vi "Turn All Outputs Off.vi"(8 "error in":errorcluster, 11 "6700C in":refnum<class "6700C.lvclass">) -> (0 "error out":errorcluster, 3 "6700C out":refnum<class "6700C.lvclass">)   [LabVIEW 2019, in "6700C.lvlib" / "6700C.lvclass"]
uses:
  Library/6700C.lvclass
  C:/Users/Public/Documents/Development/builds/Instruments/PowerSupply.lvlibp/Library/PowerSupply.lvclass
  builds/Instruments/PowerSupply.lvlibp/Private/Accessors/Read Number of Channels.vi
  builds/Instruments/PowerSupply.lvlibp/Accessors/Write Active Channel.vi
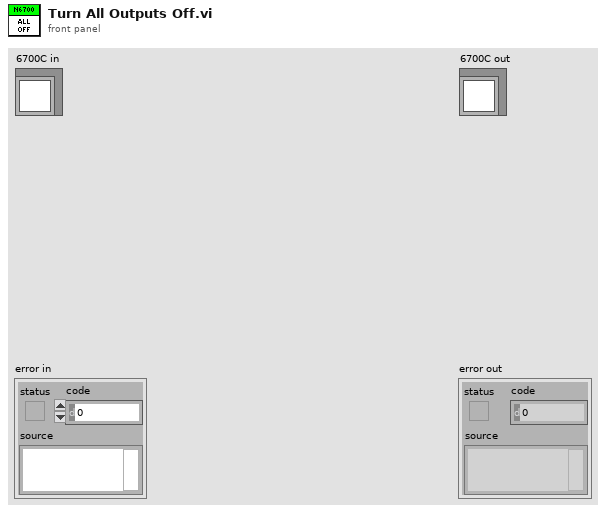
[diagram p1: front panel]
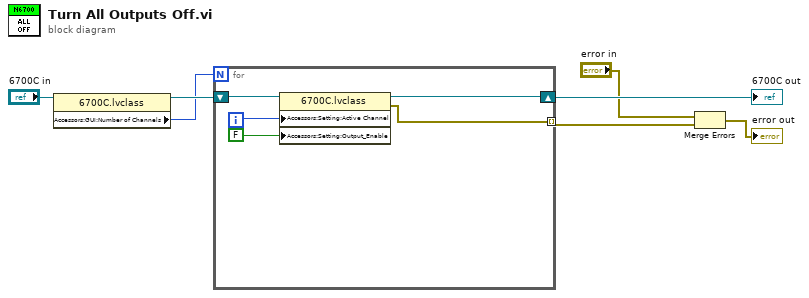
[diagram p0: block diagram]
diagram:
  n1 = property class="6700C.lvclass"(reference="6700C in") -> (reference out=w2:refnum<class "6700C.lvclass">, "Accessors:GUI:Number of Channels"=w1:i32)  [unwired: 1 in, 1 out]
  n2 = for {
    N: w1 -> [_]
    shift-right: [w9] -> w7
    shift-left: w2 -> [w12]
    tunnel: [w8] -> w6 mode=indexing
    i -> [w11]
    n3 = property class="6700C.lvclass"(reference=w12, "Accessors:Setting:Active Channel"=w11, "Accessors:Setting:Output_Enable"=FALSE ("Supply:Settings:Output_Enable")) -> (reference out=w9:refnum<class "6700C.lvclass">, error out=w8:errorcluster)  [unwired: 1 in]
  }
  "6700C out" <- w7
  n4 = Merge Errors("error in", w6) -> (→"error out":errorcluster)
